vi "StacerRangeCheck.vi"(10 "On Bert?":bool, 11 "Stacker":dbl format="%#_13g") -> (3 "In ok range to count?":bool)   [LabVIEW 2014]
panel:
  in  "Ernie Counting Ranges":T1={"Hold 4 Up Limit"=16.0, "Hold 4 Low Limit "=13.5, "Hold 5 Up Limit"=16.0, "Hold 5 Low Limit"=13.5, "Hold 6 Up Limit"=4.6, "Hold 6 Low Limit"=2.8}
  in  "Bert Counting Ranges":T1={"Hold 4 Up Limit"=16.5, "Hold 4 Low Limit "=13.5, "Hold 5 Up Limit"=16.6, "Hold 5 Low Limit"=13.5, "Hold 6 Up Limit"=4.9, "Hold 6 Low Limit"=2.8}
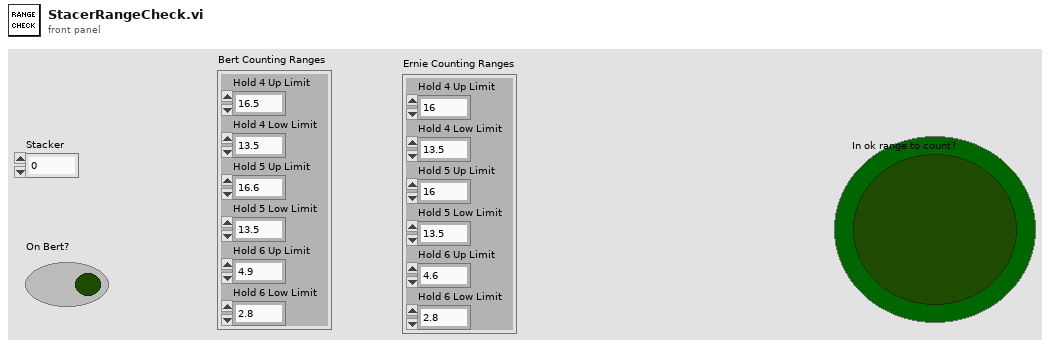
[diagram p1: front panel]
types:
  T1 = cluster{"Hold 4 Up Limit":dbl, "Hold 4 Low Limit ":dbl, "Hold 5 Up Limit":dbl, "Hold 5 Low Limit":dbl, "Hold 6 Up Limit":dbl, "Hold 6 Low Limit":dbl}
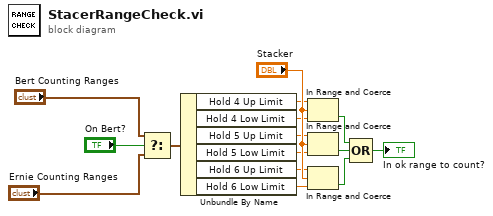
[diagram p0: block diagram]
diagram:
  n1 = Select(t="Bert Counting Ranges", s="On Bert?", f="Ernie Counting Ranges") -> (s? t:f=w7:T1)
  n2 = Unbundle By Name(w7) -> ("Hold 4 Up Limit"=w2:dbl, "Hold 4 Low Limit"=w1:dbl, "Hold 5 Up Limit"=w3:dbl, "Hold 5 Low Limit"=w4:dbl, "Hold 6 Up Limit"=w6:dbl, "Hold 6 Low Limit"=w5:dbl)
  n3 = In Range and Coerce(upper limit=w2, x="Stacker", lower limit=w1) -> (In Range?=w14:bool)  [unwired: 1 out]
  n4 = In Range and Coerce(upper limit=w3, x="Stacker", lower limit=w4) -> (In Range?=w13:bool)  [unwired: 1 out]
  n5 = In Range and Coerce(upper limit=w6, x="Stacker", lower limit=w5) -> (In Range?=w12:bool)  [unwired: 1 out]
  n6 = Compound Arithmetic op=OR(w14, w13, w12) -> (→"In ok range to count?":bool)
